vi "Which Indices.vi"(11 "In":bool[](array[boolean])) -> (3 "X":u8[](array[numeric]))   [LabVIEW 2021, in "d15.lvlib" / "Cave.lvclass"]
uses:
  Cave.lvclass
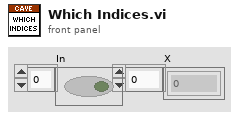
[diagram p1: front panel]
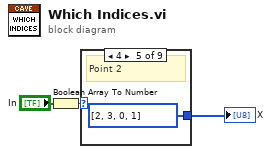
[diagram p0: block diagram]
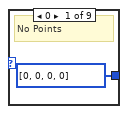
[diagram p2: hidden frame]
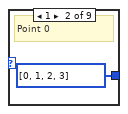
[diagram p3: hidden frame]
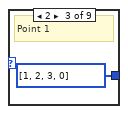
[diagram p4: hidden frame]
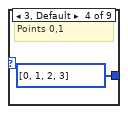
[diagram p5: hidden frame]
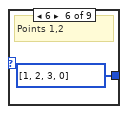
[diagram p6: hidden frame]
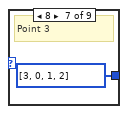
[diagram p7: hidden frame]
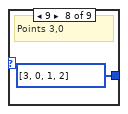
[diagram p8: hidden frame]
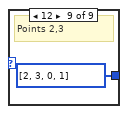
[diagram p9: hidden frame]
diagram:
  n1 = Boolean Array To Number(Boolean array="In") -> (number=w2:u32)
  n2 = case shown="4" w2 {
    tunnel: [u8[] [0, 0, 0, 0] u8[] [0, 1, 2, 3] u8[] [1, 2, 3, 0] u8[] [0, 1, 2, 3] u8[] [2, 3, 0, 1] u8[] [1, 2, 3, 0] u8[] [3, 0, 1, 2] u8[] [3, 0, 1, 2] u8[] [2, 3, 0, 1]] -> w3
    frame 0 {
      # "No Points"
    }
    frame 1 {
      # "Point 0"
    }
    frame 2 {
      # "Point 1"
    }
    frame 3, Default {
      # "Points 0,1"
    }
    frame 4 {
      # "Point 2"
    }
    frame 6 {
      # "Points 1,2"
    }
    frame 8 {
      # "Point 3"
    }
    frame 9 {
      # "Points 3,0"
    }
    frame 12 {
      # "Points 2,3"
    }
  }
  "X" <- w3
